vi "字节改动.vi"() -> ()   [LabVIEW 2017]
panel:
  out "低字节 2":u16 format="%x"
  out "高字节":u16 format="%x"
  in  "十六进制":u16 format="%x"
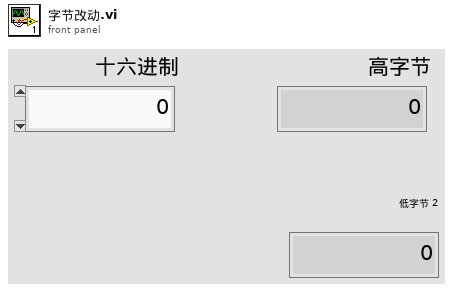
[diagram p1: front panel]
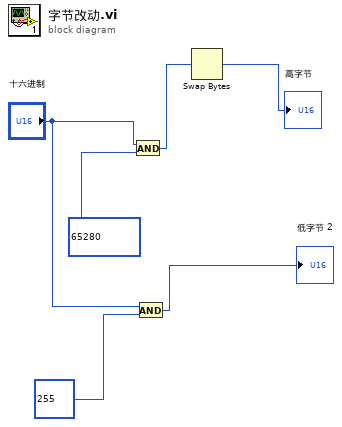
[diagram p0: block diagram]
diagram:
  n1 = And(x="十六进制", y=u16 65280) -> (x .and. y?=w2:u16)
  n2 = And(x="十六进制", y=u16 255) -> (x .and. y?=→"低字节 2":u16)
  n3 = Swap Bytes(anything=w2) -> (byte swapped=→"高字节":u16)
